vi "EZDA_JS.vi"() -> ()   [LabVIEW 2018]
panel:
  in  "stop":bool
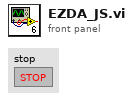
[diagram p1: front panel]
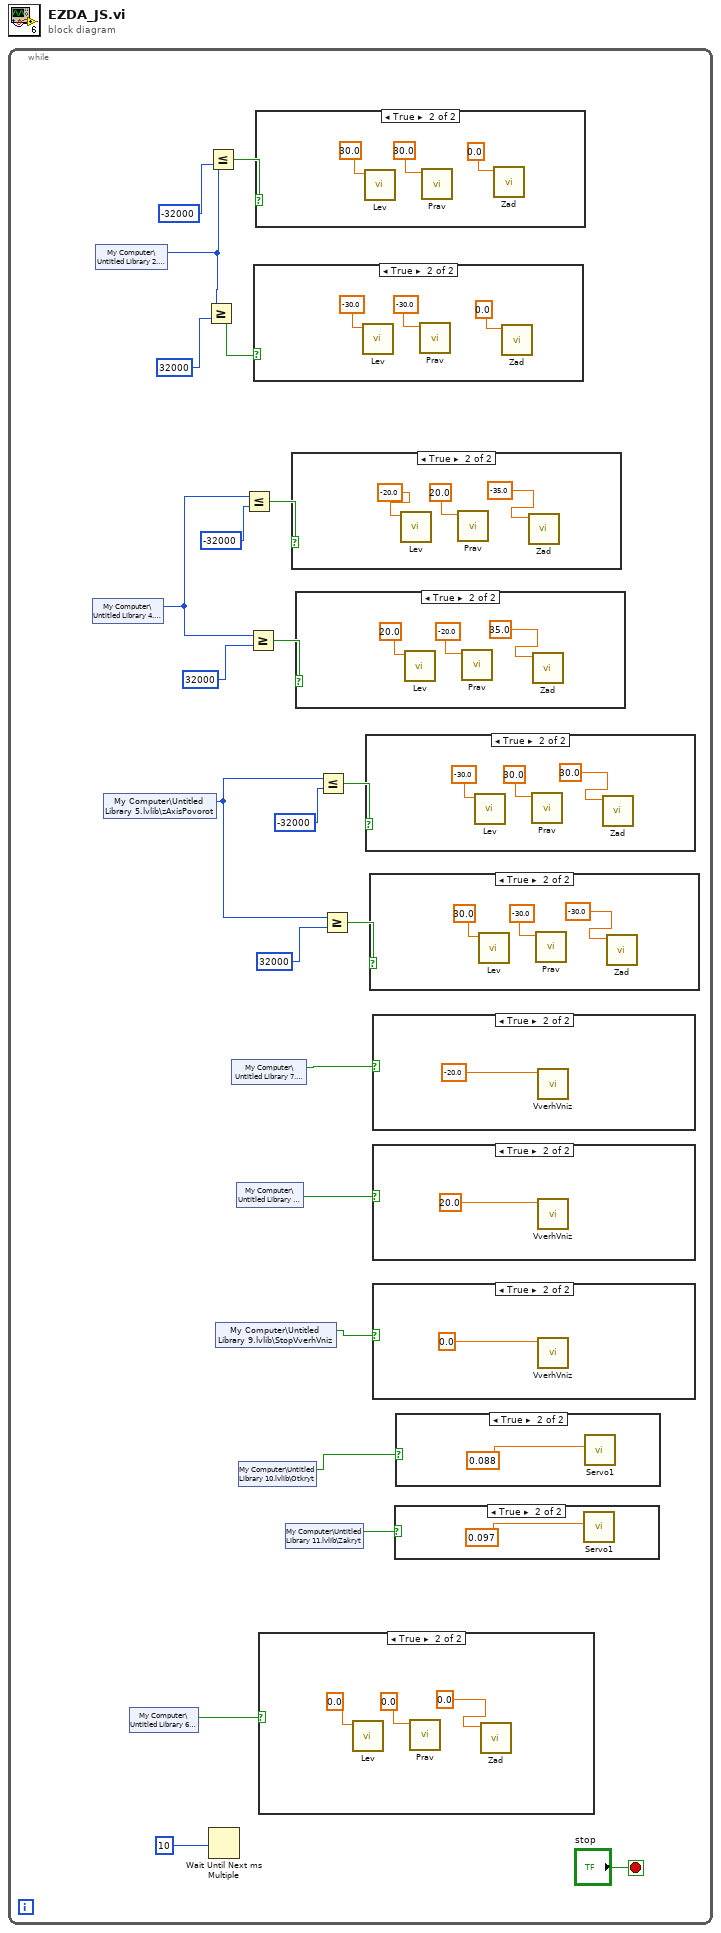
[diagram p0: block diagram]
diagram:
  n1 = while {
    stop <- "stop" stop-if-true
    n2 = shared-variable "My Computer\\Untitled Library 4.lvlib\\xAxis"() -> (w12:i32)  [unwired: 1 in, 1 out]
    n3 = shared-variable "My Computer\\Untitled Library 2.lvlib\\yAxis"() -> (w17:i32)  [unwired: 1 in, 1 out]
    n4 = shared-variable "My Computer\\Untitled Library 5.lvlib\\zAxisPovorot"() -> (w7:i32)  [unwired: 1 in, 1 out]
    n5 = shared-variable "My Computer\\Untitled Library 6.lvlib\\Stop"() -> (w6:bool)  [unwired: 1 in, 1 out]
    n6 = Greater Or Equal?(x=w17, y=32000) -> (x >= y?=w18:bool)
    n7 = Less Or Equal?(x=w17, y=-32000) -> (x <= y?=w22:bool)
    n8 = Wait Until Next ms Multiple(millisecond multiple=10) -> ()  [unwired: 1 out]
    n9 = shared-variable "My Computer\\Untitled Library 9.lvlib\\StopVverhVniz"() -> (w3:bool)  [unwired: 1 in, 1 out]
    n10 = shared-variable "My Computer\\Untitled Library 7.lvlib\\Vverh"() -> (w5:bool)  [unwired: 1 in, 1 out]
    n11 = shared-variable "My Computer\\Untitled Library 8.lvlib\\Vniz"() -> (w4:bool)  [unwired: 1 in, 1 out]
    n12 = shared-variable "My Computer\\Untitled Library 10.lvlib\\Otkryt"() -> (w2:bool)  [unwired: 1 in, 1 out]
    n13 = Less Or Equal?(x=w12, y=-32000) -> (x <= y?=w15:bool)
    n14 = Greater Or Equal?(x=w12, y=32000) -> (x >= y?=w13:bool)
    n15 = case shown="True" w18 {
      frame False {
      }
      frame True {
        n16 = call "Lev.vi"("Numeric"=-30.0) -> ()  [unwired: 9 in, 2 out]
        n17 = call "Prav.vi"("Numeric"=-30.0) -> ()  [unwired: 9 in, 2 out]
        n18 = call "Zad.vi"("Numeric"=0.0) -> ()  [unwired: 9 in, 2 out]
      }
    }
    n19 = case shown="True" w22 {
      frame False {
      }
      frame True {
        n20 = call "Lev.vi"("Numeric"=30.0) -> ()  [unwired: 9 in, 2 out]
        n21 = call "Prav.vi"("Numeric"=30.0) -> ()  [unwired: 9 in, 2 out]
        n22 = call "Zad.vi"("Numeric"=0.0) -> ()  [unwired: 9 in, 2 out]
      }
    }
    n23 = case shown="True" w6 {
      frame False {
      }
      frame True {
        n24 = call "Lev.vi"("Numeric"=0.0) -> ()  [unwired: 9 in, 2 out]
        n25 = call "Prav.vi"("Numeric"=0.0) -> ()  [unwired: 9 in, 2 out]
        n26 = call "Zad.vi"("Numeric"=0.0) -> ()  [unwired: 9 in, 2 out]
      }
    }
    n27 = shared-variable "My Computer\\Untitled Library 11.lvlib\\Zakryt"() -> (w1:bool)  [unwired: 1 in, 1 out]
    n28 = case shown="True" w15 {
      frame False {
      }
      frame True {
        n29 = call "Lev.vi"("Numeric"=-20.0) -> ()  [unwired: 9 in, 2 out]
        n30 = call "Prav.vi"("Numeric"=20.0) -> ()  [unwired: 9 in, 2 out]
        n31 = call "Zad.vi"("Numeric"=-35.0) -> ()  [unwired: 9 in, 2 out]
      }
    }
    n32 = case shown="True" w13 {
      frame False {
      }
      frame True {
        n33 = call "Lev.vi"("Numeric"=20.0) -> ()  [unwired: 9 in, 2 out]
        n34 = call "Prav.vi"("Numeric"=-20.0) -> ()  [unwired: 9 in, 2 out]
        n35 = call "Zad.vi"("Numeric"=35.0) -> ()  [unwired: 9 in, 2 out]
      }
    }
    n36 = Less Or Equal?(x=w7, y=-32000) -> (x <= y?=w10:bool)
    n37 = Greater Or Equal?(x=w7, y=32000) -> (x >= y?=w8:bool)
    n38 = case shown="True" w10 {
      frame False {
      }
      frame True {
        n39 = call "Lev.vi"("Numeric"=-30.0) -> ()  [unwired: 9 in, 2 out]
        n40 = call "Prav.vi"("Numeric"=30.0) -> ()  [unwired: 9 in, 2 out]
        n41 = call "Zad.vi"("Numeric"=30.0) -> ()  [unwired: 9 in, 2 out]
      }
    }
    n42 = case shown="True" w8 {
      frame False {
      }
      frame True {
        n43 = call "Lev.vi"("Numeric"=30.0) -> ()  [unwired: 9 in, 2 out]
        n44 = call "Prav.vi"("Numeric"=-30.0) -> ()  [unwired: 9 in, 2 out]
        n45 = call "Zad.vi"("Numeric"=-30.0) -> ()  [unwired: 9 in, 2 out]
      }
    }
    n46 = case shown="True" w5 {
      frame False {
      }
      frame True {
        n47 = call "VverhVniz.vi"("Numeric"=-20.0) -> ()  [unwired: 10 in, 1 out]
      }
    }
    n48 = case shown="True" w4 {
      frame False {
      }
      frame True {
        n49 = call "VverhVniz.vi"("Numeric"=20.0) -> ()  [unwired: 10 in, 1 out]
      }
    }
    n50 = case shown="True" w3 {
      frame False {
      }
      frame True {
        n51 = call "VverhVniz.vi"("Numeric"=0.0) -> ()  [unwired: 10 in, 1 out]
      }
    }
    n52 = case shown="True" w1 {
      frame False {
      }
      frame True {
        n53 = call "Servo1.vi"("Knob"=0.097) -> ()  [unwired: 10 in, 1 out]
      }
    }
    n54 = case shown="True" w2 {
      frame False {
      }
      frame True {
        n55 = call "Servo1.vi"("Knob"=0.088) -> ()  [unwired: 10 in, 1 out]
      }
    }
  }
